vi "init.vi"(8 "error in (no error)":errorcluster, 9 "Image Type":T1=1 items=["Grayscale (U8)", "Grayscale (I16)", "Grayscale (SGL)", "Complex (CSG)", "RGB (U32)", "HSL (U32)", "RGB (U64)", "Grayscale (U16)"], 10 "Camera Name":refnum<k21> caption="IMAQdx Session", 11 "camera in":refnum<class "camera.lvclass">) -> (0 "error out":errorcluster, 3 "camera out":refnum<class "camera.lvclass">)   [LabVIEW 2017, in "camera.lvclass"]
uses:
  camera.lvclass
  <vilib>/vision/driver/NI_Vision_Acquisition_Software.lvlib
  <resource>/objmgr/imaqdx.rc
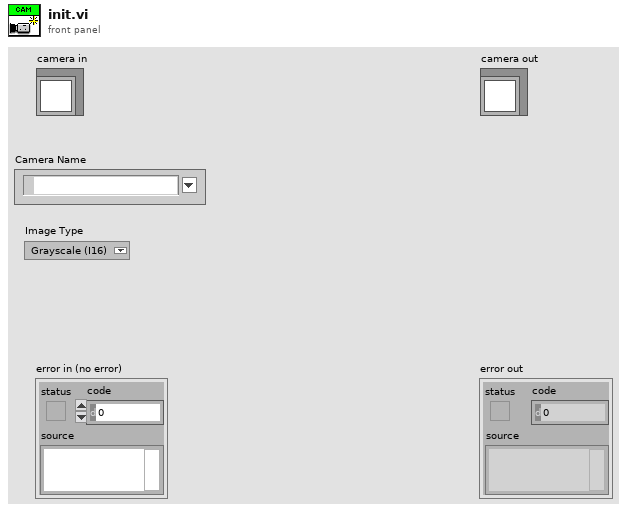
[diagram p1: front panel]
types:
  T1 = typedef "Image Type" = u32
  T2 = typedef "IMAQdx.ctl" = refnum<k21>
  T3 = typedef "IMAQ Image.ctl" = refnum<image>
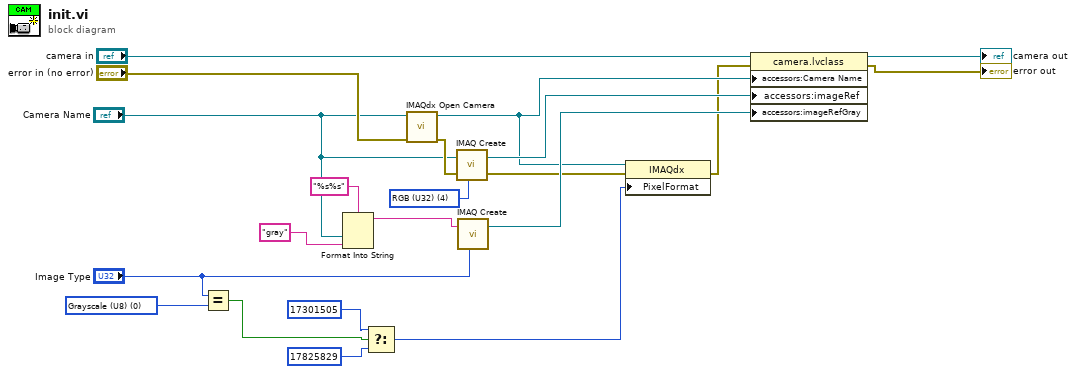
[diagram p0: block diagram]
diagram:
  w2 = T1 0 items=["Grayscale (U8)", "Grayscale (I16)", "Grayscale (SGL)", "Complex (CSG)", "RGB (U32)", "HSL (U32)", "RGB (U64)", "Grayscale (U16)"] ("Image Type 3")
  w15 = T1 4 items=["Grayscale (U8)", "Grayscale (I16)", "Grayscale (SGL)", "Complex (CSG)", "RGB (U32)", "HSL (U32)", "RGB (U64)", "Grayscale (U16)"] ("Image Type")
  n1 = Equal?(x="Image Type", y=w2) -> (x = y?=w7:bool)
  n2 = Format Into String(format string="%s%s", "Camera Name", "gray" ("Image Name")) -> (resulting string=w11:string)  [unwired: 2 in, 1 out]
  n3 = Select(t=u32 17301505 ("PixelFormat"), s=w7, f=u32 17825829 ("PixelFormat")) -> (s? t:f=w1:u32)
  n4 = call <vilib>:"IMAQdx Open Camera.vi"("error in"="error in (no error)", "Session In"="Camera Name") -> ("error out"=w19:errorcluster, "Session Out"=w9:T2)  [unwired: 1 in, 7 out]
  n5 = call "IMAQ Create"("Image Name"="Camera Name", "Image Type"=w15, "error in (no error)"=w19) -> ("New Image"=w16:T3, "error out"=w4:errorcluster)  [unwired: 1 in, 1 out]
  n6 = call "IMAQ Create"("Image Name"=w11, "Image Type"="Image Type") -> ("New Image"=w10:T3)  [unwired: 2 in, 2 out]
  n7 = property class="IMAQdx"(reference=w9, error in=w4, "PixelFormat"=w1) -> (error out=w3:errorcluster)  [unwired: 1 out]
  n8 = property class="camera.lvclass"(reference="camera in", error in=w3, "accessors:Camera Name"=w9, "accessors:imageRef"=w16, "accessors:imageRefGray"=w10) -> (reference out=→"camera out":refnum<class "camera.lvclass">, error out=→"error out":errorcluster)
